vi "readGyro.vi"() -> ()   [LabVIEW 2016]
uses:
  #defines.ctl
  AXES.ctl
  GLOBALS.vi
panel:
  out "temp":u8[](array[numeric])
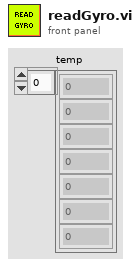
[diagram p1: front panel]
types:
  T1 = typedef "#defines.ctl" = i16
  T2 = typedef "AXES.ctl" = u16
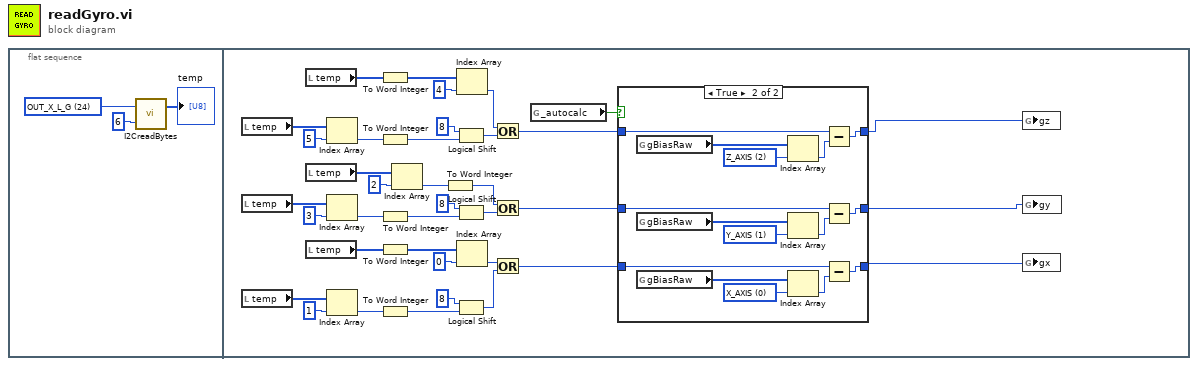
[diagram p0: block diagram]
diagram:
  n1 = flat-sequence {
    frame #0 {
      w1 = T1 24 items=["CTRL_REG9"=35, "STATUS_REG_1"=39, "OUT_X_L_XL"=40, "FIFO_CTRL"=46, "FIFO_SRC"=47, "CTRL_REG4"=30, "OUT_X_L_G"=24, "OUT_TEMP_L"=21, "INT_GEN_SRC_G"=20, "ORIENT_CFG_G"=19, "CTRL_REG3_G"=18, "CTRL_REG2_G"=17, "CTRL_REG1_G"=16, "WHO_AM_I_XG"=15] ("Ring")
      n2 = call "I2CreadBytes.vi"("count"=u8 6, "subAddress"=w1) -> ("dest"=→"temp":u8[])  [unwired: 1 out]
    }
    frame #1 {
      n3 = local read "temp"() -> (w26:u8[])
      n4 = local read "temp"() -> (w29:u8[])
      n5 = local read "temp"() -> (w33:u8[])
      n6 = local read "temp"() -> (w12:u8[])
      n7 = local read "temp"() -> (w32:u8[])
      n8 = local read "temp"() -> (w8:u8[])
      n9 = Index Array(array=w26, index=5) -> (element=w14:u8)
      n10 = Index Array(array=w29, index=3) -> (element=w18:u8)
      n11 = Index Array(array=w33, index=1) -> (element=w9:u8)
      n12 = To Word Integer(number=w12) -> (16bit integer=w11:i16[])
      n13 = To Word Integer(number=w14) -> (16bit integer=w13:i16)
      n14 = To Word Integer(number=w18) -> (16bit integer=w17:i16)
      n15 = To Word Integer(number=w8) -> (16bit integer=w7:i16[])
      n16 = To Word Integer(number=w9) -> (16bit integer=w10:i16)
      n17 = Index Array(array=w32, index=2) -> (element=w16:u8)
      n18 = To Word Integer(number=w16) -> (16bit integer=w15:i16)
      n19 = Logical Shift(y=i16 8, x=w13) -> (x << y=w37:i16)
      n20 = Logical Shift(y=i16 8, x=w17) -> (x << y=w21:i16)
      n21 = Logical Shift(y=i16 8, x=w10) -> (x << y=w38:i16)
      n22 = Index Array(array=w11, index=4) -> (element=w25:i16)
      n23 = Index Array(array=w7, index=0) -> (element=w35:i16)
      n24 = Or(x=w25, y=w37) -> (x .or. y?=w23:i16)
      n25 = Or(x=w15, y=w21) -> (x .or. y?=w19:i16)
      n26 = Or(x=w35, y=w38) -> (x .or. y?=w24:i16)
      n27 = global read "GLOBALS.vi" "_autocalc"() -> (w22:bool)
      n28 = case shown="True" w22 {
        tunnel: w24 -> [w42 w57]
        tunnel: [w42 w53] -> w6
        tunnel: [w41 w46] -> w5
        tunnel: [w43 w45] -> w4
        tunnel: w23 -> [w43 w58]
        tunnel: w19 -> [w41 w44]
        frame False {
        }
        frame True {
          w49 = T2 2 items=["X_AXIS", "Y_AXIS", "Z_AXIS", "ALL_AXIS"] ("Ring")
          w52 = T2 1 items=["X_AXIS", "Y_AXIS", "Z_AXIS", "ALL_AXIS"] ("Ring")
          w55 = T2 0 items=["X_AXIS", "Y_AXIS", "Z_AXIS", "ALL_AXIS"] ("Ring")
          n29 = global read "GLOBALS.vi" "gBiasRaw"() -> (w50:u16[])
          n30 = global read "GLOBALS.vi" "gBiasRaw"() -> (w51:u16[])
          n31 = global read "GLOBALS.vi" "gBiasRaw"() -> (w56:u16[])
          n32 = Index Array(array=w50, index=w49) -> (element=w48:u16)
          n33 = Index Array(array=w51, index=w52) -> (element=w47:u16)
          n34 = Index Array(array=w56, index=w55) -> (element=w54:u16)
          n35 = Subtract(x=w58, y=w48) -> (x-y=w45:u16)
          n36 = Subtract(x=w44, y=w47) -> (x-y=w46:u16)
          n37 = Subtract(x=w57, y=w54) -> (x-y=w53:u16)
        }
      }
      n38 = global write "GLOBALS.vi" "gz"(w4) -> ()
      n39 = global write "GLOBALS.vi" "gy"(w5) -> ()
      n40 = global write "GLOBALS.vi" "gx"(w6) -> ()
    }
  }
